vi "PH_Synchrolock_Watch.PC Reset Mira Warning.vi"(0 "i ref in":refnum<vi>, 2 "Reset Warning?":bool, 5 "error in (no error)":errorcluster) -> (14 "i ref out":refnum<vi>, 19 "error out":errorcluster)   [LabVIEW 2014, in "PH_Synchrolock_Watch.lvlib"]
doc: "This is the Proc Case \"Reset Warning\"."
uses:
  PH_Synchrolock_Watch.lvlib
  PH_Basics/PH_Common/PH_Common.lvlib
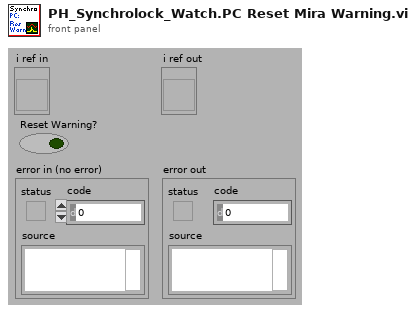
[diagram p1: front panel]
types:
  T1 = typedef "PH_Synchrolock_Watch.lvlib/PH_Synchrolock_Watch.i attribute.ctl" = cluster{"GUI Refs":cluster{"Mean Phase Graph":refnum<vi>, "RF Amplitude Graph":refnum<vi>, "Mira Amplitude Graph":refnum<vi>, "MIRA State":refnum<vi>, "Mean Phase":refnum<vi>, "RF Amplitude":refnum<vi>, "Mira Amplitude":refnum<vi>, "Mean Phase in range?":refnum<vi>, "RF Amplitude above limit?":refnum<vi>, "Mira Amplitude in range?":refnum<vi>, "Mean phase upper limit":refnum<vi>, "Mean phase lower limit":refnum<vi>, "RF Amplitude lower limit":refnum<vi>, "Mira Amplitude lower limit":refnum<vi>, "Mira Amplitude upper limit":refnum<vi>, "Waveform End":refnum<vi>, "Mira scope":refnum<vi>, "Reset Mira warning":refnum<vi>}, "Status":cluster{"Reset Warning":bool}, "Mean Phase":cluster{"Current Value":dbl, "Upper Limit":dbl, "Lower Limit":dbl, "Data":cluster{dbl[], dbl[]}}, "RF":cluster{"Current Value":dbl, "Lower Limit":dbl, "Data":cluster{dbl[], dbl[]}}, "MIRA":cluster{"Current Value":dbl, "Upper Limit":dbl, "Lower Limit":dbl, "Data":cluster{dbl[], dbl[]}}, "Waveform End":i32}
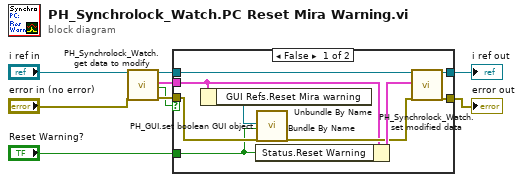
[diagram p0: block diagram]
diagram:
  n1 = call "PH_Synchrolock_Watch.get data to modify.vi"("i ref in"="i ref in", "error in (no error)"="error in (no error)") -> ("i ref out"=w9:refnum<vi>, "i attribute"=w3:T1, "timed out"=w1:bool, "error out"=w4:errorcluster)  [unwired: 14 in]
  n2 = case shown="False" w1 {
    tunnel: w9 -> [w18 w20]
    tunnel: [w17 w20] -> w6
    tunnel: [w16 w19] -> w5
    tunnel: w4 -> [w15 w19]
    tunnel: w3 -> [w12 _]
    tunnel: "Reset Warning?" -> [w10 _]
    frame False {
      n3 = Unbundle By Name(w12) -> ("GUI Refs.Reset Mira warning"=w11:refnum<vi>)
      n4 = Bundle By Name(cluster=w12, "Status.Reset Warning"=w10) -> (w14:T1)
      n5 = call "PH_GUI.set boolean GUI object.vi"("Boolean Knob GUI Ref"=w11, "Value"=w10, "error in (no error)"=w15) -> ("error out"=w13:errorcluster)  [unwired: 16 in]
      n6 = call "PH_Synchrolock_Watch.set modified data.vi"("i ref in"=w18, "i attribute"=w14, "error in (no error)"=w13) -> ("i ref out"=w17:refnum<vi>, "error out"=w16:errorcluster)  [unwired: 15 in]
    }
    frame True {
    }
  }
  "i ref out" <- w6
  "error out" <- w5
